vi "Uart write.vi"(0 "RedPitaya connection in":refnum<k5>, 1 "timeout ms (2000)":i32=2000, 9 "string to send":string, 11 "error in":errorcluster) -> (4 "RedPitaya connection out":refnum<k5>, 15 "error out":errorcluster)   [LabVIEW 2021]
uses:
  Red_Pitaya/RedPitaya.lvlib
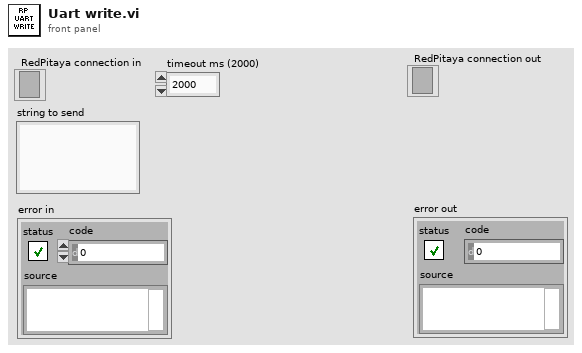
[diagram p1: front panel]
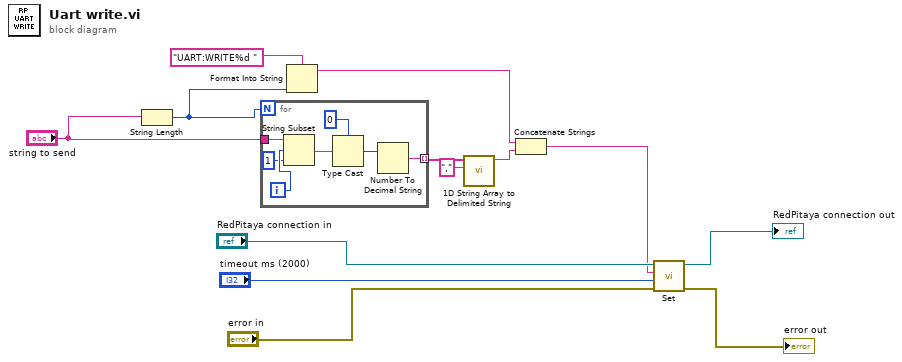
[diagram p0: block diagram]
diagram:
  n1 = String Length(string="string to send") -> (length=w1:i32)
  n2 = for {
    N: w1 -> [_]
    tunnel: "string to send" -> [w20]
    tunnel: [w14] -> w6 mode=indexing
    i -> [w19]
    n3 = String Subset(string=w20, offset (0)=w19, length (rest)=1 ("length (rest)")) -> (substring=w17:string)
    n4 = Type Cast(type=u8 0 ("length (rest)"), x=w17) -> (*(type *) &x=w15:u8)
    n5 = Number To Decimal String(number=w15) -> (decimal integer string=w14:string)  [unwired: 1 in]
  }
  n6 = Format Into String(format string="UART:WRITE%d ", w1) -> (resulting string=w3:string)  [unwired: 2 in, 1 out]
  n7 = call <vilib>:"1D String Array to Delimited String.vi"("delimiter"=",", "string array"=w6) -> ("delimited string"=w4:string)  [unwired: 9 in]
  n8 = Concatenate Strings(w3, w4) -> (w2:string)
  n9 = call "Set.vi"("error in"="error in", "timeout ms (2000)"="timeout ms (2000)", "SCPI Message"=w2, "RedPitaya connection in"="RedPitaya connection in") -> ("error out"=→"error out":errorcluster, "RedPitaya connection out"=→"RedPitaya connection out":refnum<k5>)  [unwired: 5 in, 1 out]
